vi "EAGLE Summary Dialog.vi"(10 "Table Control in":string[][](table)) -> ()   [LabVIEW 2015]
panel:
  in  "Print Button":bool
  in  "Next":bool
  out "Table Control":string[][](table)=[["Patient Number", "057235558", ""], ["Eye", "Right Eye", ""], ["Treatment Area", "Full 360", ""], ["Eye Color", "Light", ""], ["Avg. Pulse Energy", "1.4 mJ", ""], ["Number of Pulses", "100", ""], ["Time Between Pulses", "10 mSec", ""], ["Illumination Intensity", "5", ""], ["Raneging Intensity", "5", ""], ["Limbus Ring", "150", ""], ["Treatment Ring", "500 um", ""], ["Aiming Intensity", "5", ""], ["", "", ""], ["", "", ""], ["", "", ""]]
  # "4. Treatment Complete"
  # "Treatment Summary"
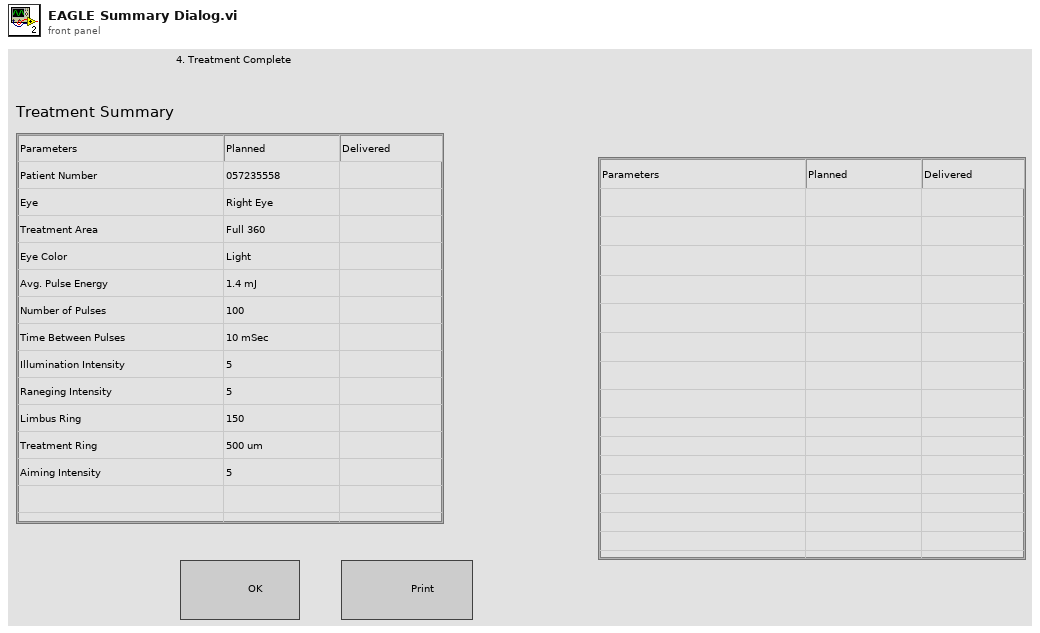
[diagram p1: front panel]
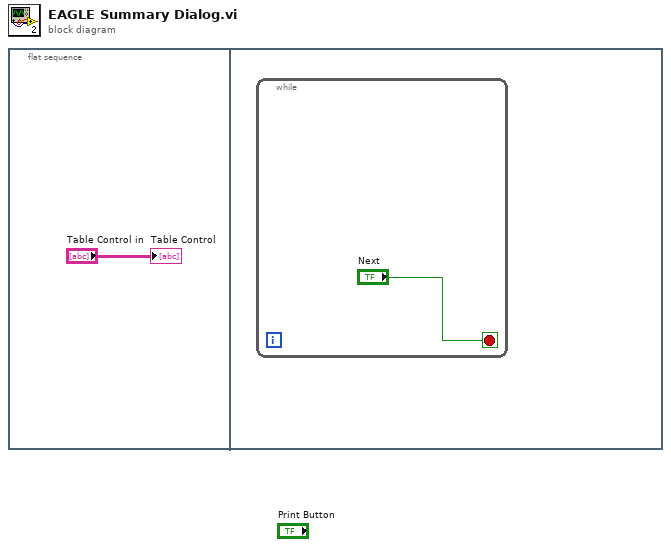
[diagram p0: block diagram]
diagram:
  n1 = flat-sequence {
    frame #0 {
      "Table Control" <- "Table Control in"
    }
    frame #1 {
      n2 = while {
        stop <- "Next" stop-if-true
      }
    }
  }
